vi "Seq Edit Step.vi"(6 "config paths":T1, 8 "Error In":errorcluster, 9 "Segment Info In":T2, 10 "Basic Steps":string[](array[string]), 11 "VI Names":string[](array[string])) -> (0 "Error Out":errorcluster, 1 "Step Hisitory":string[](array[string]), 2 "Segment Info Out":T2, 3 "Add Step?":bool)   [LabVIEW 2018]
uses:
  type defs/Sequence Info.ctl
  type defs/config paths for seq def.ctl
panel:
  out "File Name":string
  out "file or folder exists?":bool
  out "appended path":path
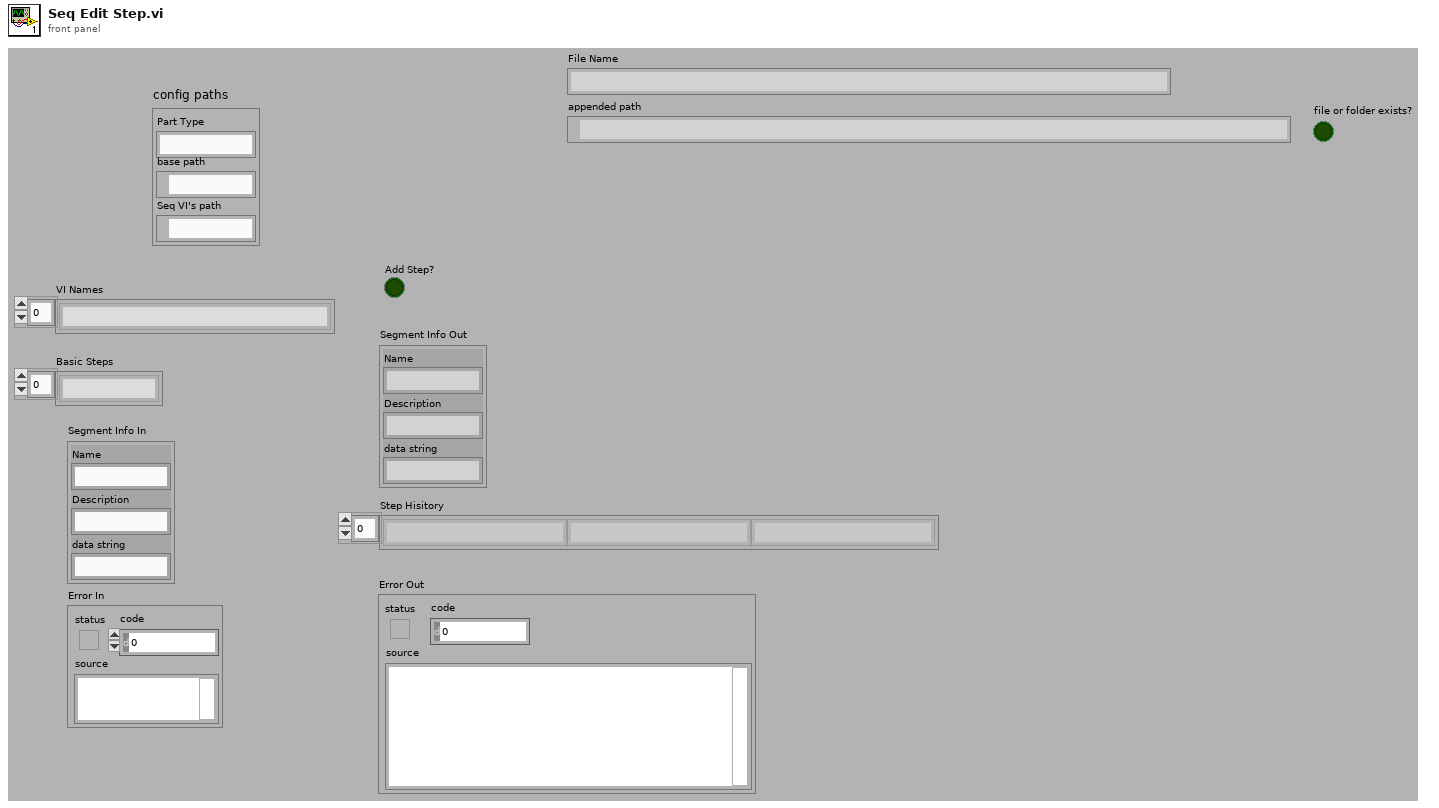
[diagram p1: front panel]
types:
  T1 = typedef "config paths for seq def.ctl" = cluster{"Part Type":string, "base path":path, "Seq VI's path":path}
  T2 = typedef "Sequence Info.ctl" = cluster{"Name":string, "Description":string, "data string":string}
  T3 = enum32{"Invalid", "Standard", "Closed", "Hidden", "Minimized", "Maximized"}
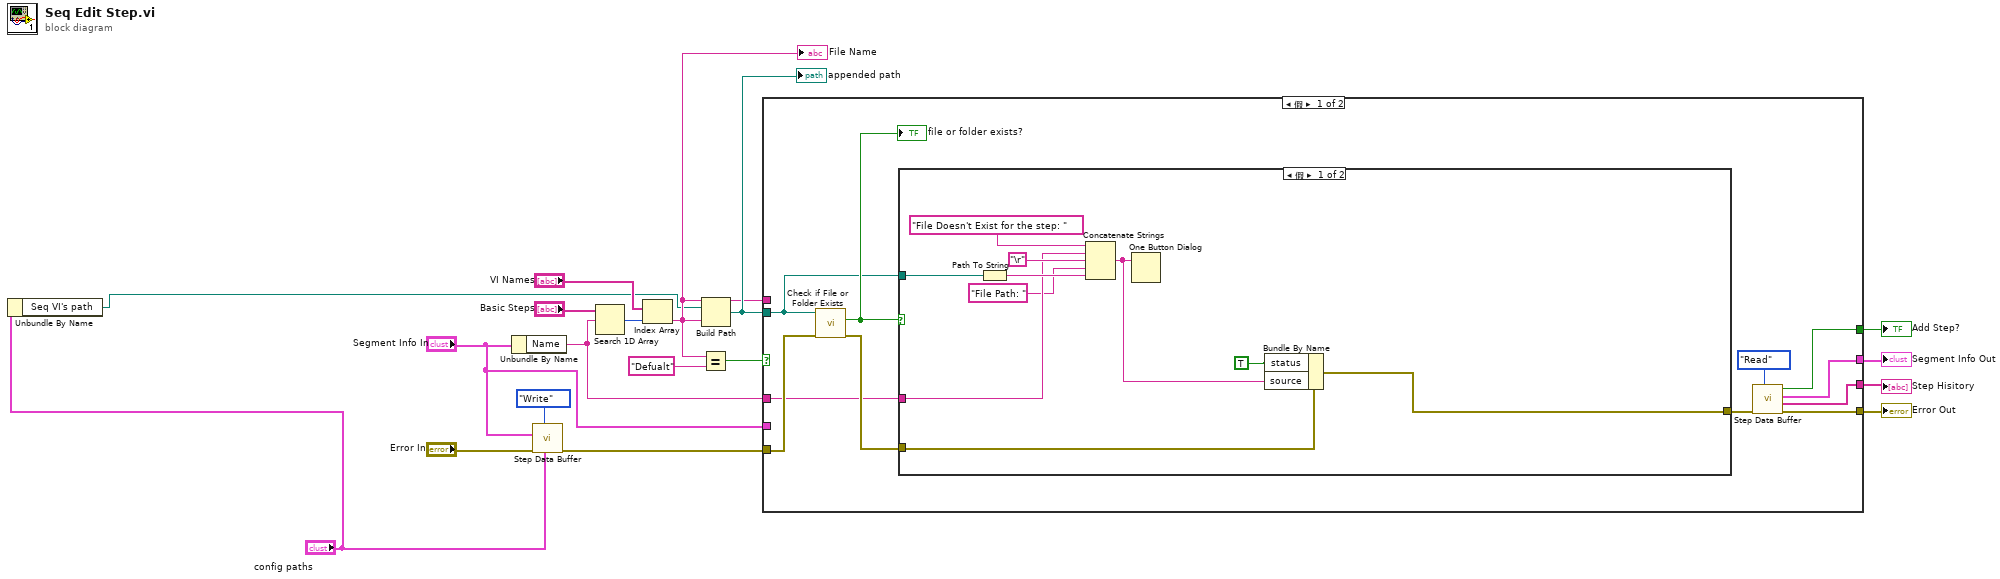
[diagram p0: block diagram]
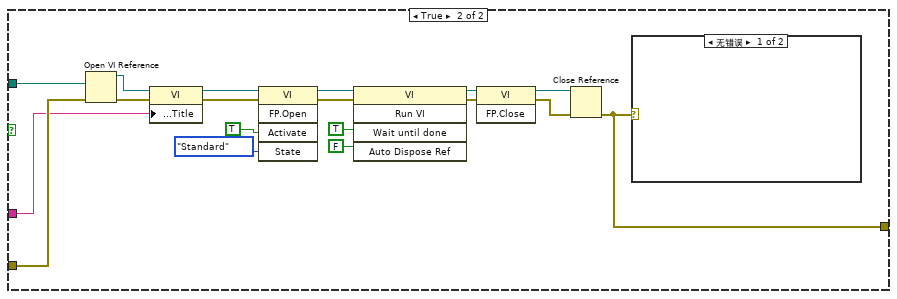
[diagram p2: hidden frame]
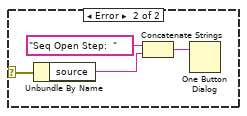
[diagram p3: hidden frame]
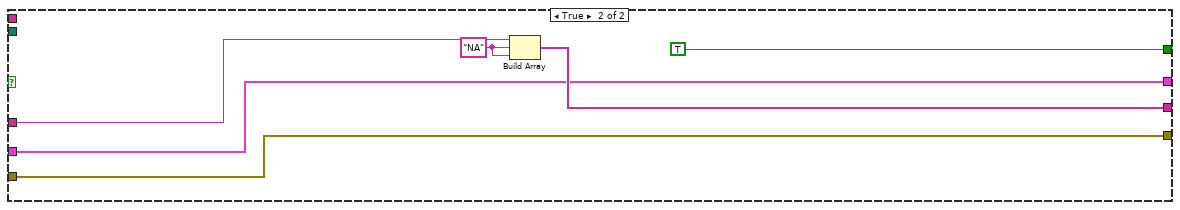
[diagram p4: hidden frame]
diagram:
  n1 = Unbundle By Name("config paths") -> ("Seq VI's path"=w1:path)
  n2 = Unbundle By Name("Segment Info In") -> ("Name"=w14:string)
  n3 = call "Step Data Buffer.vi"("config paths"="config paths", "Mode"=enum16{"Init", "Read", "Write"}."Write", "Error In"="Error In", "Segment Data"="Segment Info In") -> ("Error Out"=w11:errorcluster)  [unwired: 3 in, 4 out]
  n4 = Search 1D Array(1D array="Basic Steps", element=w14) -> (index of element=w10:i32)  [unwired: 1 in]
  n5 = Index Array(array="VI Names", index=w10) -> (element=w3:string)
  "File Name" <- w3
  n6 = Equal?(x=w3, y="Defualt") -> (x = y?=w8:bool)
  n7 = Build Path(base path=w1, name or relative path=w3) -> (appended path=w7:path)
  "appended path" <- w7
  n8 = case shown="假" w8 {
    tunnel: w7 -> [w28 _]
    tunnel: w11 -> [w27 w64]
    tunnel: [w23 w64] -> w15
    tunnel: w14 -> [w19 w66]
    tunnel: [w22 w65] -> w18
    tunnel: [w20 TRUE ("Add Step?")] -> w6
    tunnel: "Segment Info In" -> [_ w62]
    tunnel: [w21 w62] -> w4
    tunnel: w3 -> [_ _]
    frame False {
      n9 = call <vilib>:"Check if File or Folder Exists.vi"("error in (no error)"=w27, "path"=w28) -> ("error out"=w26:errorcluster, "file or folder exists?"=w29:bool)  [unwired: 7 in, 1 out]
      "file or folder exists?" <- w29
      n10 = case shown="假" w29 {
        tunnel: w28 -> [w39 w57]
        tunnel: [w32 w40] -> w24
        tunnel: w26 -> [w33 w56]
        tunnel: w19 -> [w35 w43]
        frame False {
          n11 = Path To String(path=w39) -> (string=w38:string)
          n12 = Concatenate Strings("File Doesn't Exist for the step: " ("string"), w35, "\r", "File Path: " ("string"), w38) -> (w31:string)
          n13 = One Button Dialog(message=w31) -> ()  [unwired: 1 in, 1 out]
          n14 = Bundle By Name(cluster=w33, "status"=TRUE, "source"=w31) -> (w32:errorcluster)
        }
        frame True {
          n15 = Open VI Reference(vi path=w57, error in (no error)=w56) -> (vi reference=w47:refnum<vi>, error out=w46:errorcluster)  [unwired: 4 in]
          n16 = property class="VI"(reference=w47, error in=w46, "Front Panel.Title"=w43) -> (reference out=w44:refnum<vi>, error out=w45:errorcluster)
          n17 = invoke class="VI" method="FP.Open"(reference=w44, error in=w45, "Activate"=TRUE ("Activate?"), "State"=T3."Standard") -> (reference out=w51:refnum<vi>, error out=w48:errorcluster)  [unwired: 1 in, 3 out]
          n18 = invoke class="VI" method="Run VI"(reference=w51, error in=w48, "Wait until done"=TRUE ("Wait Until Done"), "Auto Dispose Ref"=FALSE ("Auto Dispose Reference")) -> (reference out=w50:refnum<vi>, error out=w49:errorcluster)  [unwired: 1 in, 3 out]
          n19 = invoke class="VI" method="FP.Close"(reference=w50, error in=w49) -> (reference out=w42:refnum<vi>, error out=w41:errorcluster)  [unwired: 1 in, 1 out]
          n20 = Close Reference(reference=w42, error in (no error)=w41) -> (error out=w40:errorcluster)
          n21 = case shown="无错误" w40 {
            selector: w40 -> [_ w60]
            frame No Error {
            }
            frame Error {
              n22 = Unbundle By Name(w60) -> ("source"=w58:string)
              n23 = Concatenate Strings("Seq Open Step:  " ("message"), w58) -> (w59:string)
              n24 = One Button Dialog(message=w59) -> ()  [unwired: 1 in, 1 out]
            }
          }
        }
      }
      n25 = call "Step Data Buffer.vi"("Mode"=enum16{"Init", "Read", "Write"}."Read", "Error In"=w24) -> ("Error Out"=w23:errorcluster, "Step Hisitory Out"=w22:string[], "Segment Data"=w21:T2, "Add Step? Out"=w20:bool)  [unwired: 5 in, 1 out]
    }
    frame True {
      w67 = "NA" ("element")
      n26 = Build Array(w66, w67, w67) -> (w65:string[])
    }
  }
  "Step Hisitory" <- w18
  "Segment Info Out" <- w4
  "Add Step?" <- w6
  "Error Out" <- w15
